vi "SETI_Host_Interface v3.vi"() -> ()   [LabVIEW 2015]
uses:
  SETI FPGA States.ctl
  <vilib>/rvi/Emulation/niFpgaGetClockAttributes.vi
  <vilib>/rvi/Emulation/niFpgaSctlEmulationGetInTimedLoop.vi
  <vilib>/rvi/Emulation/niFpgaEmulationReportErrorSimple.vi
  <vilib>/rvi/Emulation/niFpgaProcessEmulError.vi
  <vilib>/rvi/interface/RandomDataEmulation/niFpgaRandomDataHandleErrors.vi
  <vilib>/rvi/Emulation/niFpgaCriticalErrorInLSC.vi
  <vilib>/rvi/DataTransferAndStorage/Container/XNode/niFpgaContainer.xnode
  <vilib>/rvi/interface/RandomDataEmulation/nirviRandomDataFpgaReadWriteTemplate.vi
panel:
  out "Chirp/Fft Pair 1 - Chirp Rate":fxp<+/-,64,32> format="%.42g"
  out "FPGA Loop Count":i32
  out "State":T1
  out "Total":u64
  out "Count":u64
  in  "Start":bool
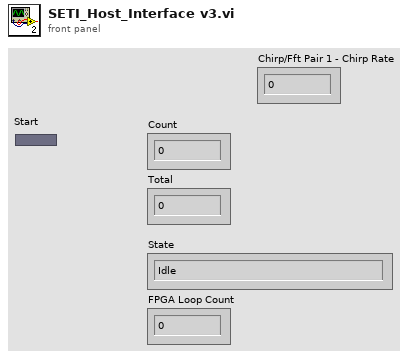
[diagram p1: front panel]
types:
  T1 = typedef "SETI FPGA States.ctl" = enum16{"Idle", "GetNumPoints", "GetChirpRate", "Process", "Stop"}
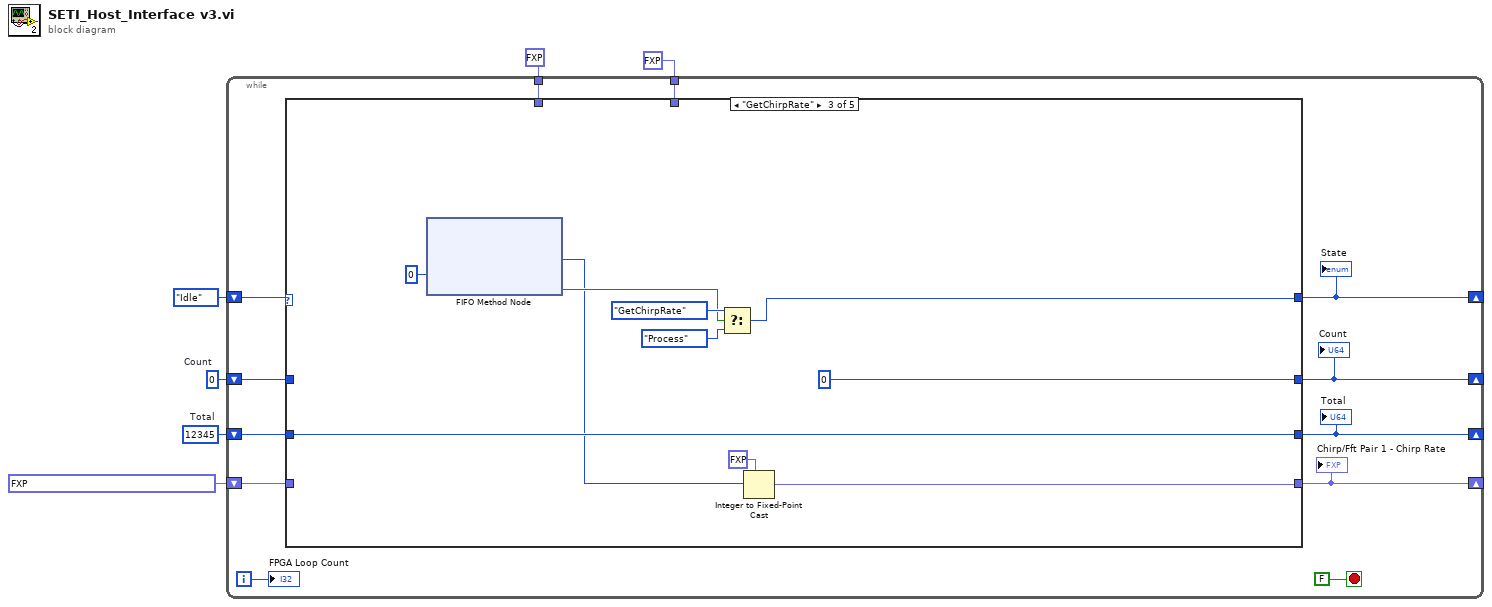
[diagram p0: block diagram]
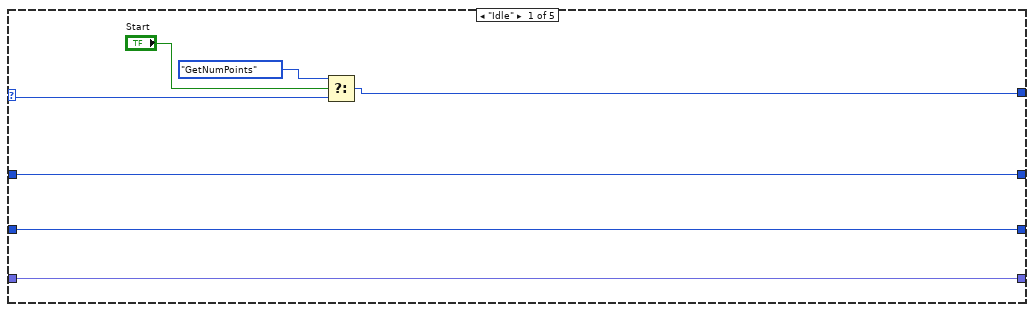
[diagram p2: hidden frame]
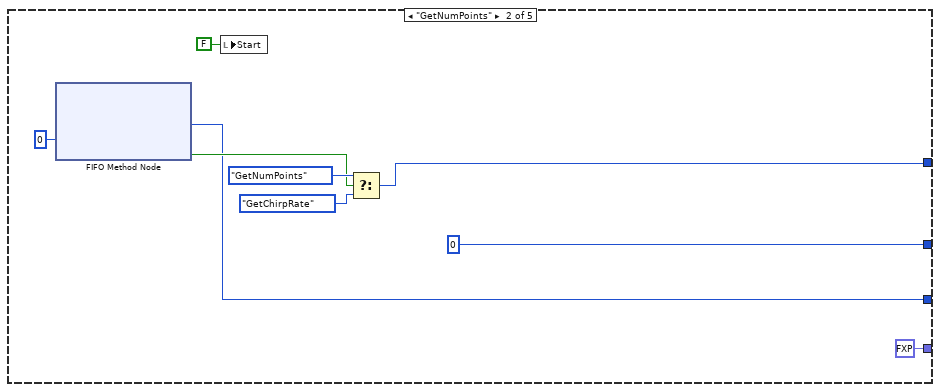
[diagram p3: hidden frame]
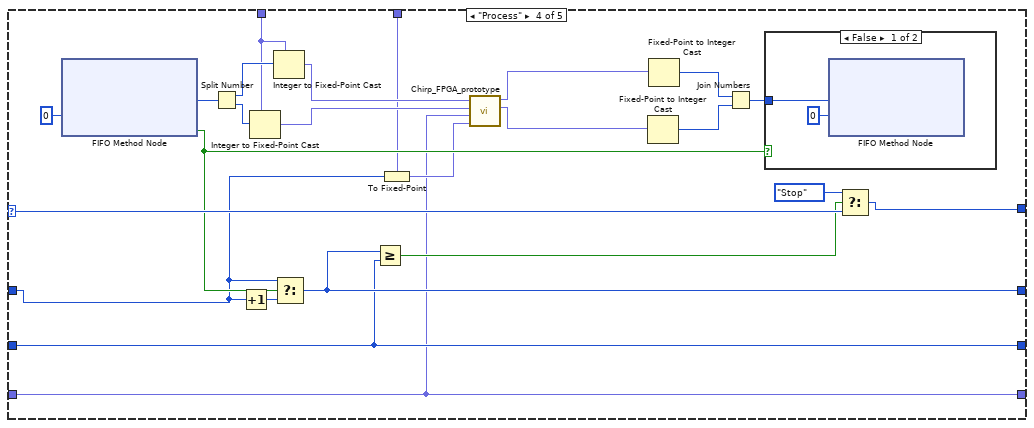
[diagram p4: hidden frame]
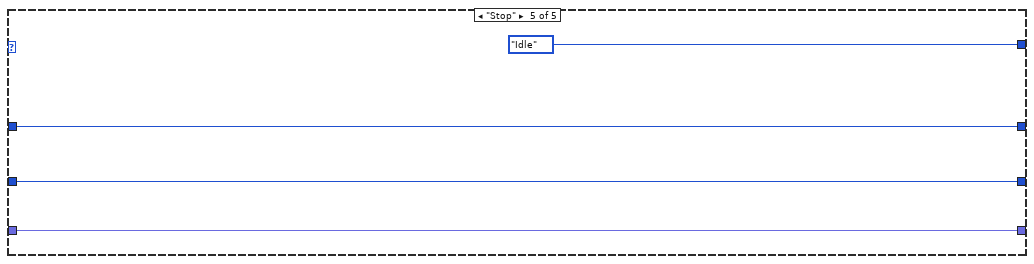
[diagram p6: hidden frame]
diagram:
  w4 = u64 12345  # Total
  w5 = u64 0  # Count
  n1 = while {
    shift-right: [w17] -> _
    shift-left: SETI_FPGA_States."Idle" -> [w18]
    shift-right: [w14] -> _
    shift-left: w5 -> [w15]
    shift-right: [w12] -> _
    shift-left: w4 -> [w13]
    tunnel: fxp<+/-,32,1> 0.0 ("real data in") -> [w10]
    tunnel: fxp<+/-,32,32> 0.0 ("Iteration") -> [w9]
    shift-right: [w7] -> _
    shift-left: fxp<+/-,64,32> 0.005545560037717223 ("Chirp/Fft Pair 1 - Chirp Rate") -> [w8]
    i -> [w11]
    stop <- FALSE stop-if-true
    n2 = case shown="\"GetChirpRate\"" w18 {
      selector: w18 -> [w24 _ _ w67 _]
      tunnel: [w23 w28 w39 w66 SETI_FPGA_States."Idle"] -> w17
      tunnel: w15 -> [w21 _ _ w48 w73]
      tunnel: [w21 u64 0 ("Timeout") u64 0 ("Timeout") w62 w73] -> w14
      tunnel: w13 -> [w20 _ w38 w61 w72]
      tunnel: [w20 w27 w38 w61 w72] -> w12
      tunnel: w10 -> [_ _ _ w53 _]
      tunnel: w9 -> [_ _ _ w46 _]
      tunnel: w8 -> [w19 _ _ w45 w71]
      tunnel: [w19 fxp<+/-,64,32> 0.0 ("Chirp/Fft Pair 1 - Chirp Rate") w36 w45 w71] -> w7
      frame "Idle" {
        n3 = Select(t=SETI_FPGA_States."GetNumPoints", s="Start", f=w24) -> (s? t:f=w23:T1)
      }
      frame "GetNumPoints" {
        n4 = xnode ("FIFO Method Node")("Timeout"=0) -> ("Element"=w27:u64, "Timed Out?"=w30:bool)  [unwired: 1 in, 1 out]
        n5 = local write "Start"(FALSE ("Start")) -> ()
        n6 = Select(t=SETI_FPGA_States."GetNumPoints", s=w30, f=SETI_FPGA_States."GetChirpRate") -> (s? t:f=w28:T1)
      }
      frame "GetChirpRate" {
        n7 = xnode ("FIFO Method Node")("Timeout"=0) -> ("Element"=w37:u64, "Timed Out?"=w41:bool)  [unwired: 1 in, 1 out]
        n8 = Select(t=SETI_FPGA_States."GetChirpRate", s=w41, f=SETI_FPGA_States."Process") -> (s? t:f=w39:T1)
        n9 = Integer to Fixed-Point Cast(fixed-point type=fxp<+/-,64,32> 0.0 ("Chirp/Fft Pair 1 - Chirp Rate"), integer=w37) -> (fixed-point=w36:fxp<+/-,64,32>)
      }
      frame "Process" {
        n10 = xnode ("FIFO Method Node")("Timeout"=0) -> ("Element"=w54:u64, "Timed Out?"=w60:bool)  [unwired: 1 in, 1 out]
        n11 = Split Number(x=w54) -> (hi(x)=w58:u32, lo(x)=w59:u32)
        n12 = Increment(x=w48) -> (x+1=w63:u64)
        n13 = Integer to Fixed-Point Cast(fixed-point type=w53, integer=w59) -> (fixed-point=w49:fxp<+/-,32,1>)
        n14 = Integer to Fixed-Point Cast(fixed-point type=w53, integer=w58) -> (fixed-point=w52:fxp<+/-,32,1>)
        n15 = Select(t=w48, s=w60, f=w63) -> (s? t:f=w62:u64)
        n16 = Greater Or Equal?(x=w62, y=w61) -> (x >= y?=w65:bool)
        n17 = To Fixed-Point(fixed-point type=w46, number=w48) -> (fixed-point=w47:fxp<+/-,32,32>)
        n18 = call "Chirp_FPGA_prototype.vi"("Iteration"=w47, "Chirp/Fft Pair 1 - Chirp Rate"=w45, "Imaginary In"=w49, "Real In"=w52) -> ("Imaginary Out"=w50:fxp<+/-,64,2>, "Real Out"=w51:fxp<+/-,64,2>)  [unwired: 6 in]
        n19 = Fixed-Point to Integer Cast(1:w50) -> (0:w56:i64)
        n20 = Fixed-Point to Integer Cast(1:w51) -> (0:w57:i64)
        n21 = Join Numbers(hi=w57, lo=w56) -> ((hi.lo)=w55:u64)
        n22 = case shown="False" w60 {
          tunnel: w55 -> [w70 _]
          frame False {
            n23 = xnode ("FIFO Method Node")("Element"=w70, "Timeout"=0) -> ()  [unwired: 1 in, 2 out]
          }
          frame True {
          }
        }
        n24 = Select(t=SETI_FPGA_States."Stop", s=w65, f=w67) -> (s? t:f=w66:T1)
      }
      frame "Stop" {
      }
    }
    "Count" <- w14
    "Total" <- w12
    "State" <- w17
    "Chirp/Fft Pair 1 - Chirp Rate" <- w7
    "FPGA Loop Count" <- w11
  }
